vi "force_clamp_v2.vi"(4 "handle in":i32, 6 "Pos 0":dbl, 7 "Desired Force (pN)":dbl, 8 "error in (no error)":errorcluster, 9 "BT":dbl, 10 "Apply Force":bool, 11 "x":dbl) -> (0 "error out":errorcluster, 3 "Numeric out":dbl)   [LabVIEW 2019]
uses:
  <vilib>/addons/control/pid/pid.llb/PID (DBL).vi
  <vilib>/addons/control/pid/NI_PID_pid.lvlib
  controller/SubVIs_nanostage/Madlib.dll
panel:
  in  "PID gains":T1={"proportional gain (Kc)"=20.0, "integral time (Ti, min)"=0.008, "derivative time (Td, min)"=0.001} {"derivative time (Td, min)" format="%.3f"; "integral time (Ti, min)" format="%.3f"; "proportional gain (Kc)" format="%.3f"}
  # "PID for holding a tethered DNA molecule ata constant force, determined by the BT value of the QPD.\nThe code is mainly inspired by the PID example VI shipped with LabVIEW. See it for further details."
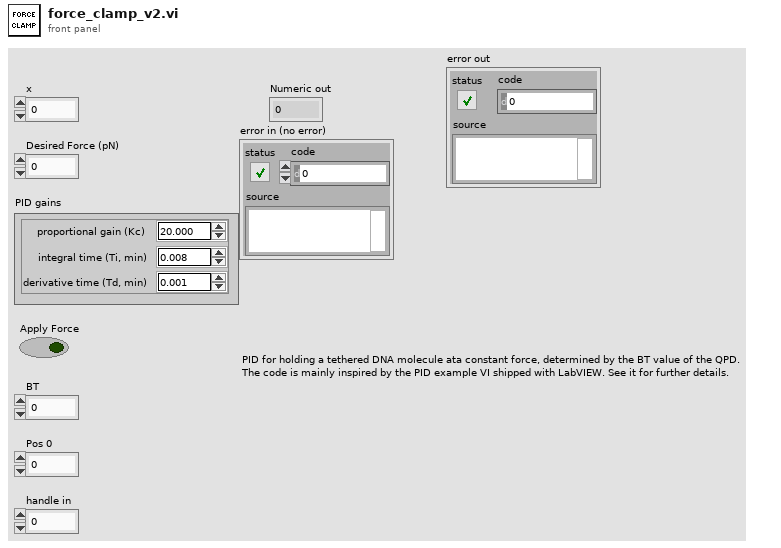
[diagram p1: front panel]
types:
  T1 = cluster{"proportional gain (Kc)":dbl, "integral time (Ti, min)":dbl, "derivative time (Td, min)":dbl}
  T2 = cluster{"static gain":dbl, "lag (min)":dbl, "dead cycles":dbl, "load %":dbl, "deadband":dbl, "noise level %":dbl, "initial PV":dbl, "initial PV 2":dbl}
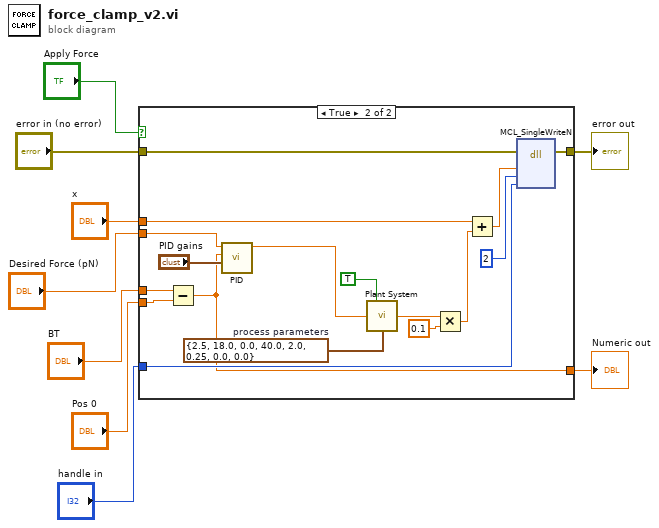
[diagram p0: block diagram]
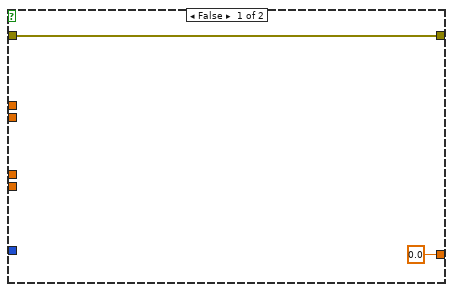
[diagram p2: hidden frame]
diagram:
  n1 = case shown="True" "Apply Force" {
    tunnel: "BT" -> [_ w28]
    tunnel: "Pos 0" -> [_ w18]
    tunnel: "Desired Force (pN)" -> [_ w17]
    tunnel: [0.0 w12] -> w7
    tunnel: "x" -> [_ w16]
    tunnel: "handle in" -> [_ w15]
    tunnel: "error in (no error)" -> [w10 w14]
    tunnel: [w10 w13] -> w1
    frame False {
    }
    frame True {
      w25 = T2 {"static gain"=2.5, "lag (min)"=18.0, "dead cycles"=0.0, "load %"=40.0, "deadband"=2.0, "noise level %"=0.25, "initial PV"=0.0, "initial PV 2"=0.0}  # process parameters
      n2 = Subtract(x=w28, y=w18) -> (x-y=w12:dbl)
      n3 = call-poly <vilib>:"PID.vi"("PID gains"="PID gains", "process variable"=w12, "setpoint"=w17) -> ("output"=w26:dbl)  [unwired: 7 in, 1 out]
      n4 = call "Plant System.vi"("Integrator ?"=TRUE, "Plant Input"=w26, "process parameters"=w25) -> ("Plant Output"=w22:dbl)  [unwired: 12 in]
      n5 = Multiply(x=w22, y=0.1) -> (x*y=w21:dbl)
      n6 = Add(x=w16, y=w21) -> (x+y=w20:dbl)
      n7 = dll-call lib="C:/Users/admin/Desktop/controller/SubVIs_nanostage/MADLib.dll" fn="MCL_SingleWriteN"(error in=w14, "position"=w20, "axis"=u32 2, "handle"=w15) -> (error out=w13:errorcluster)  [unwired: 6 in, 1 out]
    }
  }
  "Numeric out" <- w7
  "error out" <- w1
